vi "calculateLFromVAndW.vi"(8 "v_tang_curve":dbl, 9 "v_ang_curve":dbl, 10 "angle":dbl) -> (3 "L":dbl)   [LabVIEW 2023, in "Game.lvclass"]
uses:
  Game.lvclass
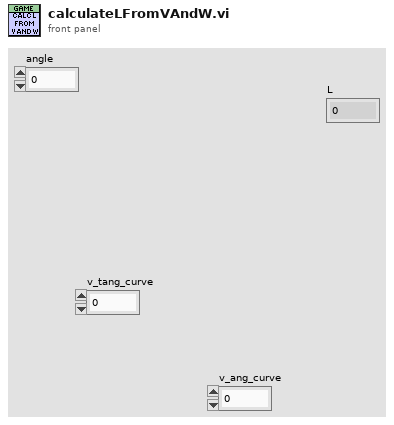
[diagram p1: front panel]
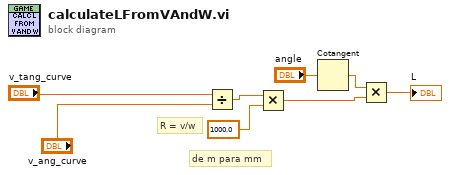
[diagram p0: block diagram]
diagram:
  # "de m para mm"
  # "R = v/w"
  n1 = Divide(x="v_tang_curve", y="v_ang_curve") -> (x/y=w5:dbl)
  n2 = Multiply(x=w5, y=1000.0) -> (x*y=w6:dbl)
  n3 = Cotangent(1:"angle") -> (0:w3:dbl)
  n4 = Multiply(x=w3, y=w6) -> (x*y=→"L":dbl)
